vi "VNA_Data_Read.vi"() -> ()   [LabVIEW 2017]
panel:
  out "Numeric":dbl
  out "Waveform Chart":dbl[](graph)
  out "error out":errorcluster
  out "VISA VNA Out":refnum<visa-resource-name>
  in  "VISA resource in":refnum<visa-resource-name>
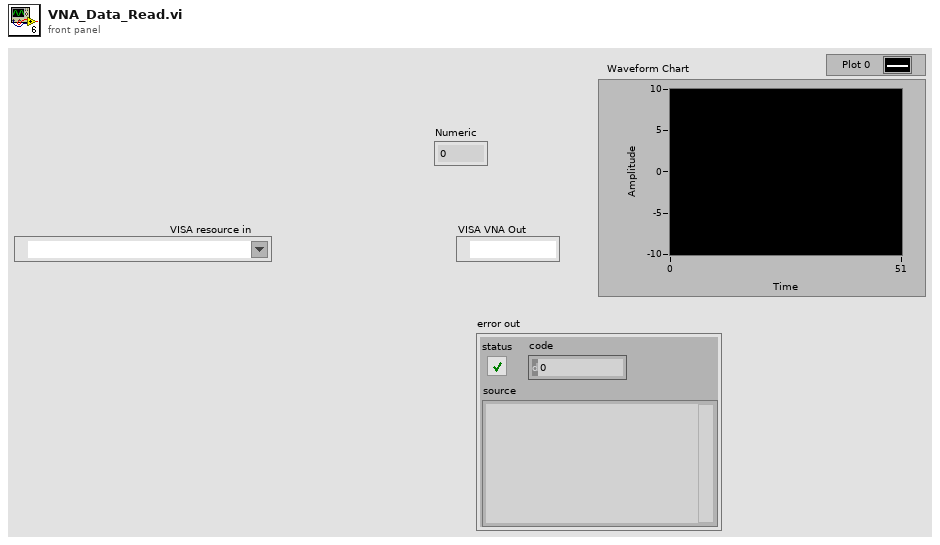
[diagram p1: front panel]
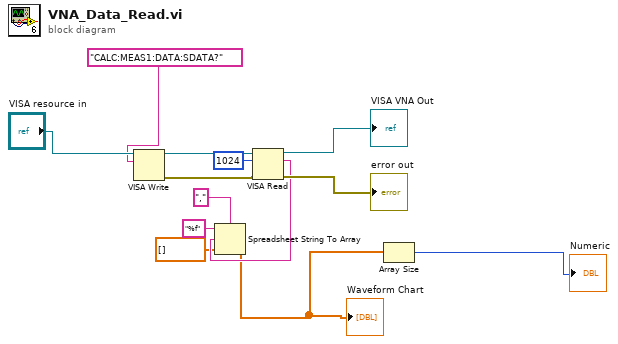
[diagram p0: block diagram]
diagram:
  n1 = VISA Write(VISA resource name="VISA resource in", write buffer="CALC:MEAS1:DATA:SDATA?") -> (VISA resource name out=w11:refnum<visa-resource-name>, error out=w9:errorcluster)  [unwired: 1 in, 1 out]
  n2 = VISA Read(VISA resource name=w11, byte count=u32 1024, error in (no error)=w9) -> (VISA resource name out=→"VISA VNA Out":refnum<visa-resource-name>, read buffer=w6:string, error out=→"error out":errorcluster)  [unwired: 1 out]
  n3 = Spreadsheet String To Array(delimiter (Tab)=",", format string="%f", spreadsheet string=w6, array type (2D Dbl)=dbl[] []) -> (array=w1:dbl[])
  "Waveform Chart" <- w1
  n4 = Array Size(array=w1) -> (size(s)=→"Numeric":i32)
